vi "DMM_Get Attributes.vi"(8 "error in (no error)":errorcluster, 11 "3446X in":refnum<class "3446X.lvclass">) -> (0 "error out":errorcluster, 2 "Class Attributes":T1, 3 "3446X out":refnum<class "3446X.lvclass">)   [LabVIEW 2015, in "3446X.lvclass"]
uses:
  3446X.lvclass
  Controls/Class Attributes Cluster.ctl
  3446X.lvclass/3446X.ctl
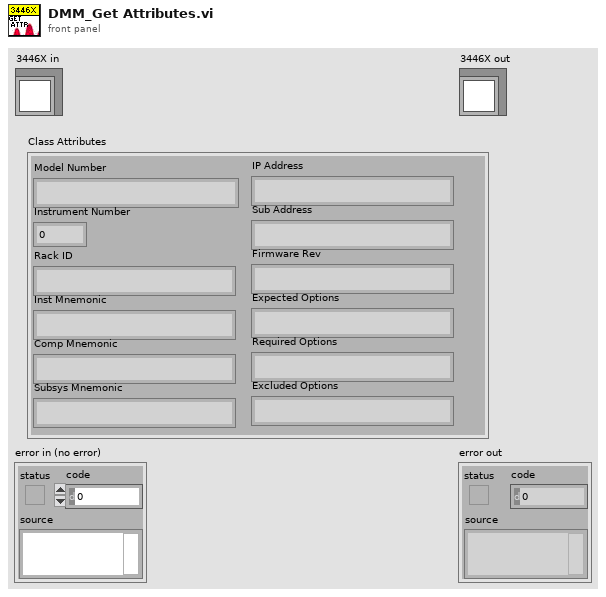
[diagram p1: front panel]
types:
  T1 = typedef "Class Attributes Cluster.ctl" = cluster{"Model Number":string, "Instrument Number":u8, "Rack ID":string, "Inst Mnemonic":string, "Comp Mnemonic":string, "Subsys Mnemonic":string, "IP Address":string, "Sub Address":string, "Firmware Rev":string, "Expected Options":string, "Required Options":string, "Excluded Options":string}
  T2 = typedef "Class Instrument Info.ctl" = string[]
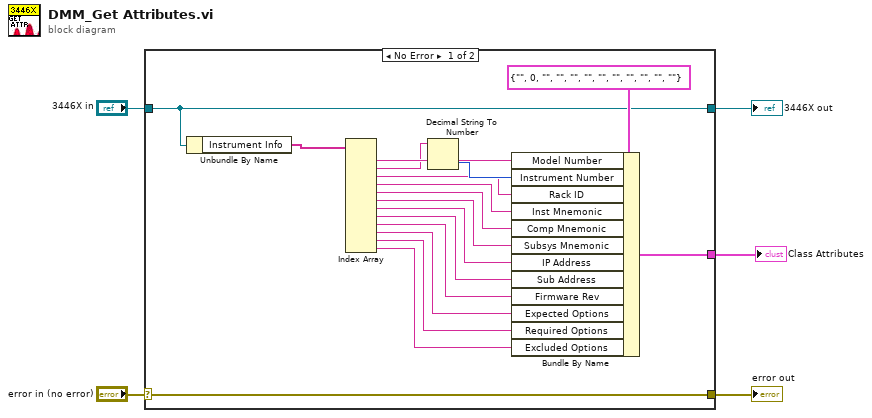
[diagram p0: block diagram]
diagram:
  n1 = case shown="No Error" "error in (no error)" {
    selector: "error in (no error)" -> [w23 w25]
    tunnel: [w23 w25] -> w3
    tunnel: [w7 w24] -> w1
    tunnel: "3446X in" -> [w7 w24]
    tunnel: [w6 _] -> w2
    frame No Error {
      n2 = Unbundle By Name(w7) -> ("Instrument Info"=w22:T2)
      n3 = Index Array(array=w22) -> (element #1=w20:string, element #2=w19:string, element #3=w17:string, element #4=w16:string, element #5=w15:string, element #6=w14:string, element #7=w13:string, element #8=w12:string, element #9=w11:string, element #10=w10:string, element #11=w9:string, element #12=w8:string)  [unwired: 12 in]
      n4 = Decimal String To Number(string=w19) -> (number=w18:i32)  [unwired: 2 in, 1 out]
      n5 = Bundle By Name(cluster=T1 {"Model Number"="", "Instrument Number"=0, "Rack ID"="", "Inst Mnemonic"="", "Comp Mnemonic"="", "Subsys Mnemonic"="", "IP Address"="", "Sub Address"="", "Firmware Rev"="", "Expected Options"="", "Required Options"="", "Excluded Options"=""} ("Class Attributes"), "Model Number"=w20, "Instrument Number"=w18, "Rack ID"=w17, "Inst Mnemonic"=w16, "Comp Mnemonic"=w15, "Subsys Mnemonic"=w14, "IP Address"=w13, "Sub Address"=w12, "Firmware Rev"=w11, "Expected Options"=w10, "Required Options"=w9, "Excluded Options"=w8) -> (w6:T1)
    }
    frame Error {
    }
  }
  "error out" <- w3
  "3446X out" <- w1
  "Class Attributes" <- w2
